vi "MethodNotImplemented.vi"(8 "error in (no error)":errorcluster, 11 "LabVIEW Object In":refnum<class>) -> (0 "error out":errorcluster)   [LabVIEW 2014]
doc: "Use this to generate an informative error for an abstract method being called without being overridden in child"
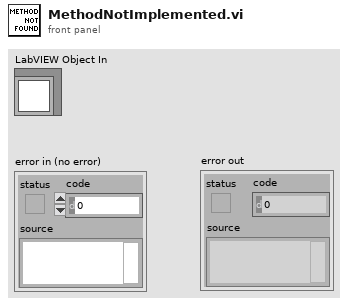
[diagram p1: front panel]
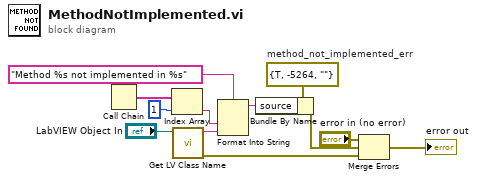
[diagram p0: block diagram]
diagram:
  w12 = errorcluster {"status"=TRUE, "code"=-5264, "source"=""}  # method_not_implemented_err
  n1 = Call Chain() -> (call chain=w11:string[])
  n2 = Index Array(array=w11, index=1) -> (element=w8:string)
  n3 = call "Get LV Class Name.vi"("object"="LabVIEW Object In") -> ("error out"=w5:errorcluster, "class name"=w6:string)  [unwired: 9 in]
  n4 = Format Into String(format string="Method %s not implemented in %s", w8, w6) -> (resulting string=w7:string)  [unwired: 2 in, 1 out]
  n5 = Bundle By Name(cluster=w12, "source"=w7) -> (w4:errorcluster)
  n6 = Merge Errors("error in (no error)", w4, w5) -> (→"error out":errorcluster)
